vi "I2C Temperature Humidity Sensor DH20.vi"() -> ()   [LabVIEW 2020, in "CTI-Scratchpad.lvlib"]
uses:
  CTI-Scratchpad.lvlib
  CTI/Identity.ctl
  CTI/Error Reporting.ctl
  CTI/GPIO Number.ctl
  CTI/I2C Number.ctl
  CTI/Session/Session.lvclass
  CTI-Peripheral/Analog Input/Grove I2C Sensors/Temperature and Humidity/Grove Temperature Humidity Sensor DH20.lvclass
  CTI/VisaComms/VisaComms.lvclass
  CTI/CTI.lvlib
panel:
  out "Humidity 2":dbl(slide) scale=0.0..100.0
  out "Thermometer":dbl(slide) scale=0.0..100.0
  out "Humidity":dbl(graph)
  out "Temperature":dbl(graph)
  in  "Stop":bool
  out "loop":i32
  out "Identity":T1
  in  "Grove Connector":enum16{"I2C0", "I2C1"}(ring)
  out "error out":errorcluster
  in  "Port":refnum<visa-resource-name>="COM4"
  # "https://wiki.seeedstudio.com/Grove-Temperature-Humidity-Sensor-DH20/"
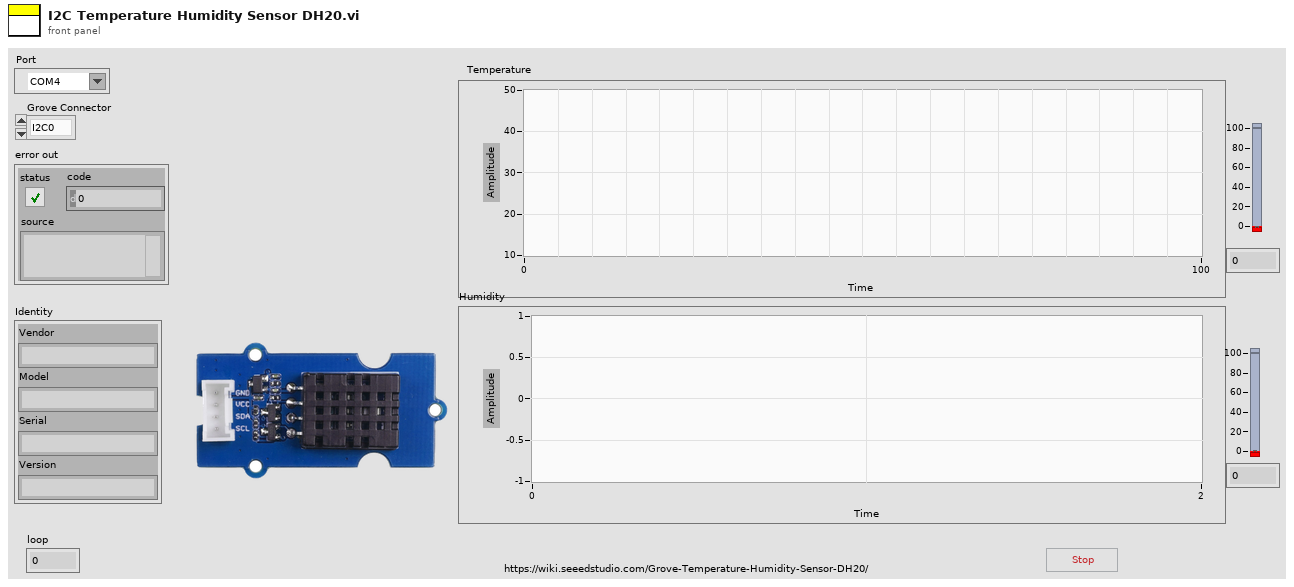
[diagram p1: front panel]
types:
  T1 = typedef "CTI.lvlib/Identity.ctl" = cluster{"Vendor":string, "Model":string, "Serial":string, "Version":string}
  T2 = typedef "CTI.lvlib/Error Reporting.ctl" = enum16{"Minimal", "Moderate", "Full"}
  T3 = typedef "CTI.lvlib/I2C Number.ctl" = i8
  T4 = typedef "CTI.lvlib/GPIO Number.ctl" = i8
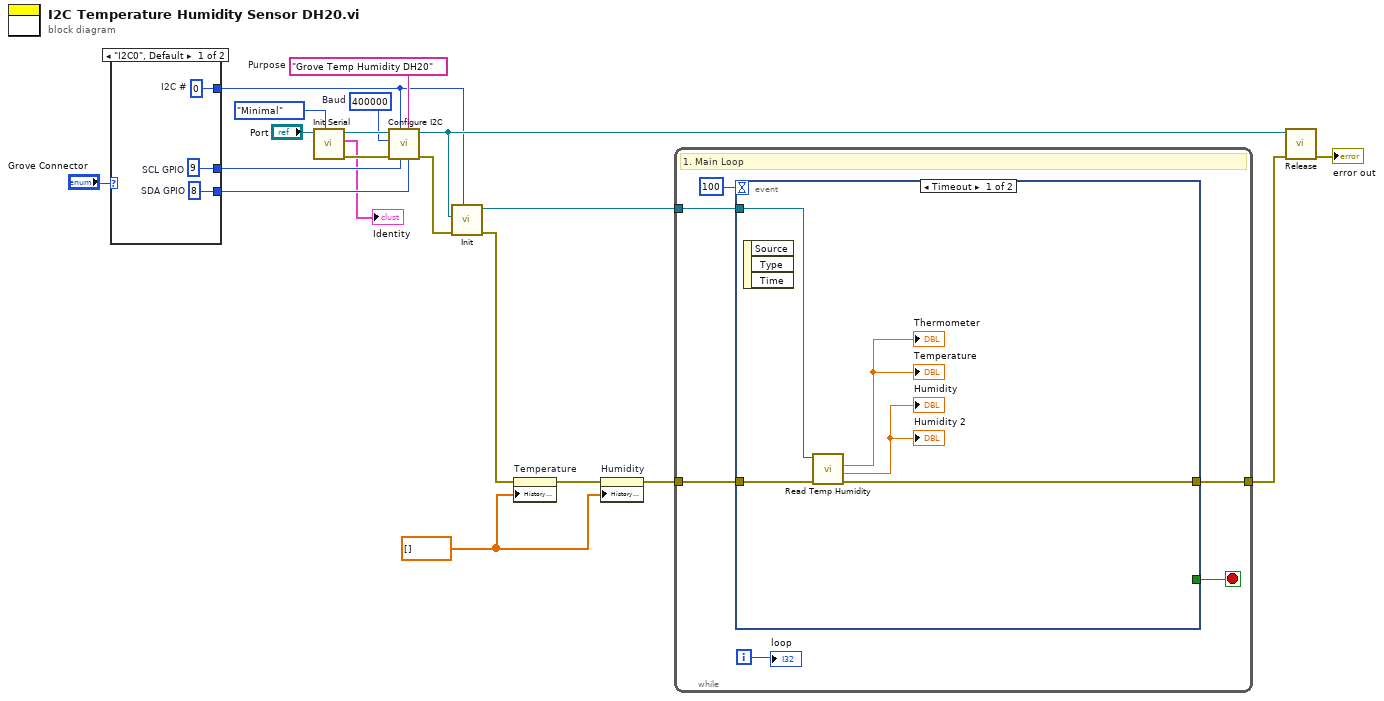
[diagram p0: block diagram]
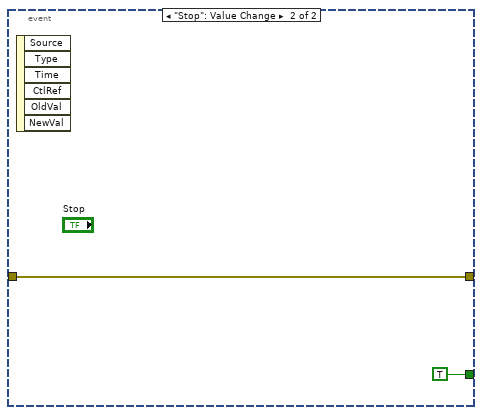
[diagram p2: hidden frame]
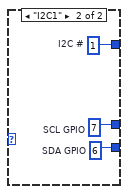
[diagram p3: hidden frame]
diagram:
  w3 = dbl[] [] ("History Data")
  w15 = "Grove Temp Humidity DH20"  # Purpose
  w16 = u32 400000  # Baud
  n1 = case shown="\"I2C0\", Default" "Grove Connector" {
    tunnel: [w23 w26] -> w11
    tunnel: [w22 w25] -> w10
    tunnel: [w21 w24] -> w9
    frame "I2C0", Default {
      w21 = T3 0  # I2C #
      w22 = T4 8  # SDA GPIO
      w23 = T4 9  # SCL GPIO
    }
    frame "I2C1" {
      w24 = T3 1  # I2C #
      w25 = T4 6  # SDA GPIO
      w26 = T4 7  # SCL GPIO
    }
  }
  n2 = call "Init Serial.vi"("Error Checking (Full)"=Error_Reporting."Minimal", "VISA resource name in"="Port") -> ("error out"=w17:errorcluster, "Identity"=→"Identity":T1, "Session"=w18:refnum<class "Session.lvclass">)  [unwired: 7 in]
  n3 = call "Configure I2C.vi"("SDA GPIO"=w10, "Purpose (\"I2C\")"=w15, "SCL GPIO"=w11, "I2C #"=w9, "error in (no error)"=w17, "Baud"=w16, "Session in"=w18) -> ("error out"=w14:errorcluster, "Session out"=w13:refnum<class "Session.lvclass">)  [unwired: 3 in]
  n4 = call "Init.vi"("I2C #"=w9, "error in (no error)"=w14, "Session In"=w13) -> ("error out"=w4:errorcluster, "Grove Temperature Humidity Sensor DH20 Out"=w7:refnum<class "Grove Temperature Humidity Sensor DH20.lvclass">)  [unwired: 7 in]
  n5 = property on="Temperature" class="WFChart (strict)"(error in=w4, "History Data"=w3) -> (error out=w2:errorcluster)  [unwired: 1 in, 1 out]
  n6 = property on="Humidity" class="WFChart (strict)"(error in=w2, "History Data"=w3) -> (error out=w1:errorcluster)  [unwired: 1 in, 1 out]
  n7 = while {
    tunnel: w1 -> [w31]
    tunnel: w7 -> [w32]
    tunnel: [w29] -> w6
    i -> [w30]
    stop <- w27 stop-if-true
    # "1. Main Loop"
    n8 = event shown="[0] Timeout" {
      selector: _ -> [_ _]
      dyn-events: _ -> [_ _]
      timeout: 100 -> [_ _]
      tunnel: w32 -> [w36 _]
      tunnel: w31 -> [w37 w38]
      tunnel: [w34 w38] -> w29
      tunnel: [_ TRUE] -> w27
      event Timeout {
        n9 = event-data() -> ()  [unwired: 1 in, 3 out]
        n10 = call-dynamic "Read Temp Humidity.vi"("error in (no error)"=w37, "Grove Temperature Humidity Sensor DH20 in"=w36) -> ("error out"=w34:errorcluster, "Humidity"=→"Humidity" →"Humidity 2":dbl, "Temperature"=→"Temperature" →"Thermometer":dbl)  [unwired: 6 in, 1 out]
      }
      event "Stop": Value Change {
        n11 = event-data() -> ()  [unwired: 1 in, 6 out]
      }
    }
    "loop" <- w30
  }
  n12 = call-dynamic "Release.vi"("error in (no error)"=w6, "Session in"=w13) -> ("error out"=→"error out":errorcluster)  [unwired: 9 in]
